vi "Header Table.vi"(5 "Cell Configuration":T1={"Cell Defaults"={"Background Color"=16777215, "Horizontal Align"=3, "Vertical Align"=1, "Minimum Height"=0.0, "Fixed Height"=0.0, "Padding"={"Left"=2.0, "Top"=2.0, "Right"=2.0, "Bottom"=3.0}}, "Borders"={"Left"={"Enabled"=FALSE, "Width"=1.0, "Color"=0}, "Top"={"Enabled"=FALSE, "Width"=1.0, "Color"=0}, "Right"={"Enabled"=FALSE, "Width"=1.0, "Color"=0}, "Bottom"={"Enabled"=FALSE, "Width"=1.0, "Color"=0}}, "Column Span"=0} {"Cell Defaults"."Vertical Align" items=["Bottom", "Middle", "Top"]; "Cell Defaults"."Horizontal Align" items=["Center", "Justified", "JustifiedAll", "Left", "Right"]}, 6 "Font":T6={"Font"="Arial", "Size"=10, "Colour"=0, "Bold"=FALSE, "Italic"=FALSE, "Underline"=FALSE, "Strikethrough"=FALSE, "Font Encoding"=enum."Cp1252, WinANSI"}, 7 "Table Configuration":T4={"Table Settings"={"Number of Columns"=2, "Width (%)"=100.0, "Relative Column Widths (%)"=[50.0, 50.0], "Horizontal Align"=0, "Header Rows"=0}, "Cell Defaults"={"Background Color"=16777215, "Horizontal Align"=3, "Vertical Align"=1, "Minimum Height"=0.0, "Fixed Height"=0.0, "Padding"={"Left"=2.0, "Top"=2.0, "Right"=2.0, "Bottom"=3.0}}, "Borders"={"Left"={"Enabled"=FALSE, "Width"=1.0, "Color"=16777215}, "Top"={"Enabled"=FALSE, "Width"=1.0, "Color"=16777215}, "Right"={"Enabled"=FALSE, "Width"=1.0, "Color"=16777215}, "Bottom"={"Enabled"=FALSE, "Width"=1.0, "Color"=16777215}, "Middle Horizontal"={"Enabled"=FALSE, "Width"=0.5, "Color"=16777215}, "Middle Vertical"={"Enabled"=FALSE, "Width"=0.5, "Color"=16777215}}} {"Cell Defaults"."Vertical Align" items=["Bottom", "Middle", "Top"]; "Cell Defaults"."Horizontal Align" items=["Center", "Justified", "JustifiedAll", "Left", "Right"]; "Table Settings"."Horizontal Align" items=["Center"=0, "Left"=3, "Right"=4]}, 8 "error in":errorcluster, 9 "Column Ratio left":sgl[](array[numeric]), 10 "Table":string[][](array[string]), 11 "Context In":refnum<class "Context.lvclass">=refnum) -> (0 "error out":errorcluster, 3 "Context Out":refnum<class "Context.lvclass">)   [LabVIEW 2020, in "PDF Interface.lvlib" / "PDF Interface Helper.lvlib"]
uses:
  PDF Interface Helper.lvlib
  <vilib>/Simplicity AI/SAI_PDF_API/Classes/Context/Controls/SAI_PDF_Font.ctl
  <vilib>/Simplicity AI/SAI_PDF_API/Classes/Context/Controls/SAI_PDF_Font Encoding.ctl
  <vilib>/Simplicity AI/SAI_PDF_API/Classes/Table Builder/Controls/SAI_PDF_Table Configuration.ctl
  <vilib>/Simplicity AI/SAI_PDF_API/Classes/Table Builder/Controls/SAI_PDF_Table Horizontal Align.ctl
  <vilib>/Simplicity AI/SAI_PDF_API/Classes/Table Builder/Controls/SAI_PDF_Default Cell Format.ctl
  <vilib>/Simplicity AI/SAI_PDF_API/Classes/Table Builder/Controls/SAI_PDF_BorderLine.ctl
  <vilib>/Simplicity AI/SAI_PDF_API/Classes/Table Builder/Controls/SAI_PDF_Cell Configuration.ctl
  <vilib>/Simplicity AI/SAI_PDF_API/Classes/Context/Context.lvclass
  <vilib>/Simplicity AI/SAI_PDF_API/Classes/Table Builder/Table Builder.lvclass
  Linearisierung V2/SpanEinstellungen/SpanEinstellungen.lvlib
panel:
  # "(Cp1252)"
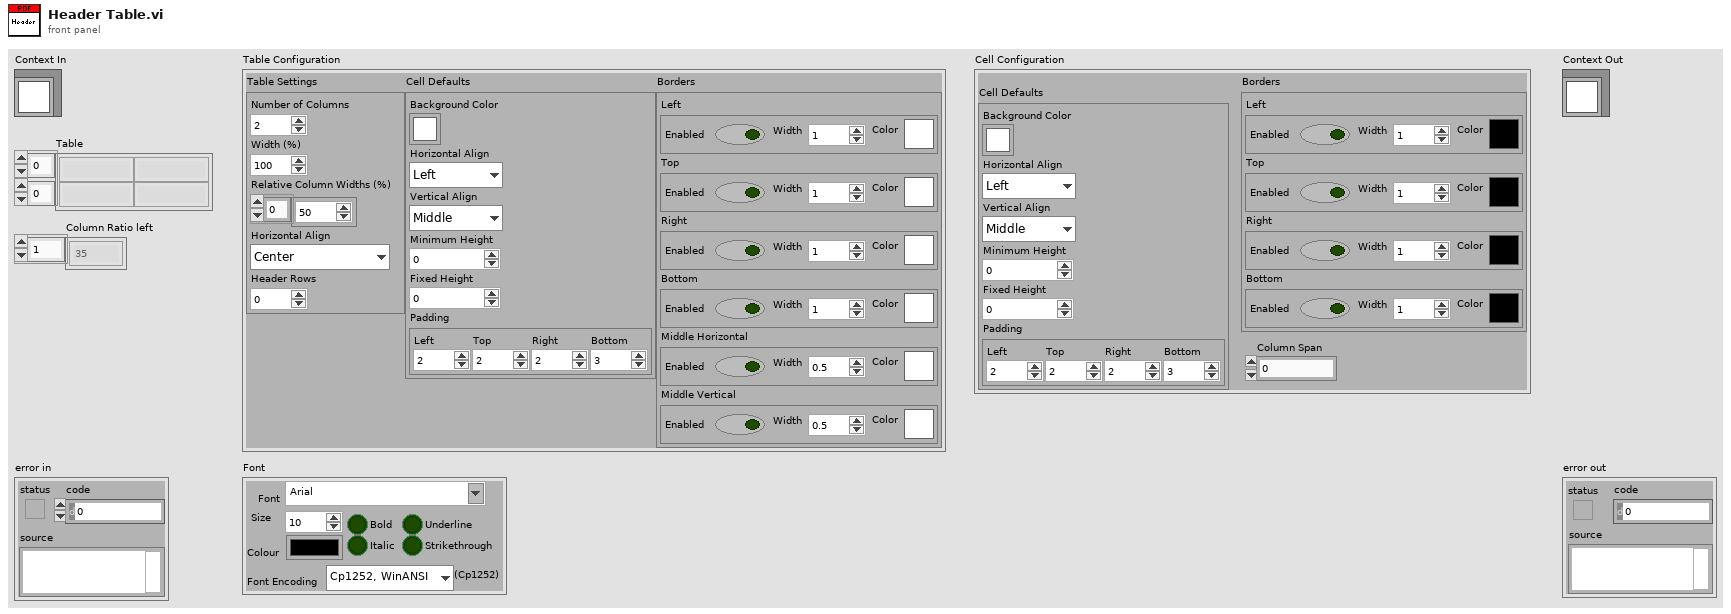
[diagram p1: front panel]
types:
  T1 = typedef "SAI_PDF_Toolkit.lvlib/Table Builder.lvclass/SAI_PDF_Cell Configuration.ctl" = cluster{"Cell Defaults":T2, "Borders":cluster{"Left":T3, "Top":T3, "Right":T3, "Bottom":T3}, "Column Span":i32}
  T2 = typedef "SAI_PDF_Toolkit.lvlib/Table Builder.lvclass/SAI_PDF_Default Cell Format.ctl" = cluster{"Background Color":u32, "Horizontal Align":i32, "Vertical Align":i32, "Minimum Height":sgl, "Fixed Height":sgl, "Padding":cluster{"Left":sgl, "Top":sgl, "Right":sgl, "Bottom":sgl}}
  T3 = typedef "SAI_PDF_Toolkit.lvlib/Table Builder.lvclass/SAI_PDF_BorderLine.ctl" = cluster{"Enabled":bool, "Width":sgl, "Color":u32}
  T4 = typedef "SAI_PDF_Toolkit.lvlib/Table Builder.lvclass/SAI_PDF_Table Configuration.ctl" = cluster{"Table Settings":cluster{"Number of Columns":i32, "Width (%)":sgl, "Relative Column Widths (%)":sgl[], "Horizontal Align":T5, "Header Rows":i32}, "Cell Defaults":T2, "Borders":cluster{"Left":T3, "Top":T3, "Right":T3, "Bottom":T3, "Middle Horizontal":T3, "Middle Vertical":T3}}
  T5 = typedef "SAI_PDF_Toolkit.lvlib/Table Builder.lvclass/SAI_PDF_Table Horizontal Align.ctl" = i32
  T6 = typedef "SAI_PDF_Toolkit.lvlib/Context.lvclass/SAI_PDF_Font.ctl" = cluster{"Font":string, "Size":i32, "Colour":u32, "Bold":bool, "Italic":bool, "Underline":bool, "Strikethrough":bool, "Font Encoding":T7}
  T7 = typedef "SAI_PDF_Toolkit.lvlib/Context.lvclass/SAI_PDF_Font Encoding.ctl" = enum16{"Cp1252, WinANSI", "IdentityH", "IdentityV", "Cp1250", "Cp1257", "MacRoman"}
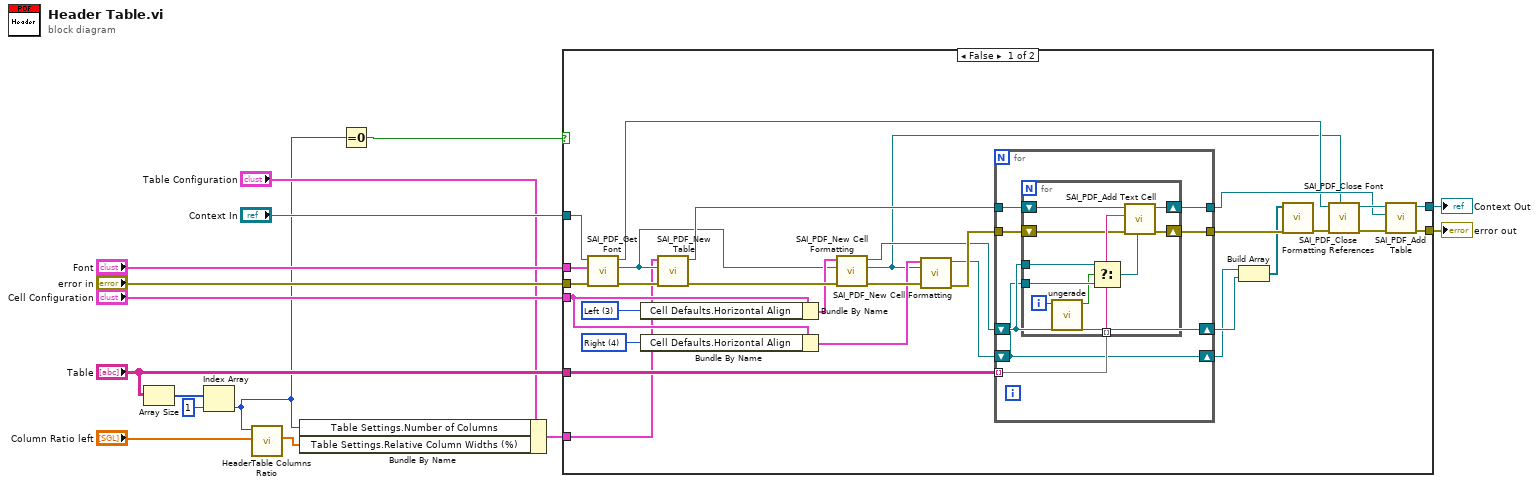
[diagram p0: block diagram]
diagram:
  n1 = Array Size(array="Table") -> (size(s)=w8:i32[])
  n2 = Index Array(array=w8, index=1 ("Index")) -> (element=w2:i32)
  n3 = call "HeaderTable Columns Ratio.vi"("Ratio left"="Column Ratio left", "Numerisch"=w2) -> ("Array ratio"=w4:sgl[])  [unwired: 8 in, 1 out]
  n4 = Bundle By Name(cluster="Table Configuration", "Table Settings.Number of Columns"=w2, "Table Settings.Relative Column Widths (%)"=w4) -> (w5:T4)
  n5 = Equal To 0?(x=w2) -> (x = 0?=w1:bool)
  n6 = case shown="False" w1 {
    tunnel: "Font" -> [w44 _]
    tunnel: "error in" -> [w43 w62]
    tunnel: "Context In" -> [w42 w63]
    tunnel: "Cell Configuration" -> [w36 _]
    tunnel: [w20 w63] -> w11
    tunnel: [w19 w62] -> w10
    tunnel: "Table" -> [w17 _]
    tunnel: w5 -> [w16 _]
    frame False {
      w40 = 4 items=["Center", "Justified", "JustifiedAll", "Left", "Right"] ("Horizontal Align")
      w39 = 3 items=["Center", "Justified", "JustifiedAll", "Left", "Right"] ("Horizontal Align")
      n7 = call <vilib>:"SAI_PDF_Get Font.vi"("error in"=w43, "Font"=w44, "Context In"=w42) -> ("error out"=w41:errorcluster, "Font"=w18:refnum<class "Font.lvclass">, "Context Out"=w21:refnum<class "Context.lvclass">)  [unwired: 6 out]
      n8 = Bundle By Name(cluster=w36, "Cell Defaults.Horizontal Align"=w39) -> (w37:T1)
      n9 = Bundle By Name(cluster=w36, "Cell Defaults.Horizontal Align"=w40) -> (w34:T1)
      n10 = call <vilib>:"SAI_PDF_New Table.vi"("error in"=w41, "Font In"=w18, "Table Configuration"=w16) -> ("error out"=w38:errorcluster, "Table Builder"=w33:refnum<class "Table Builder.lvclass">)  [unwired: 7 out]
      n11 = call <vilib>:"SAI_PDF_New Cell Formatting.vi"("error in"=w38, "Font In"=w18, "Cell Configuration"=w37) -> ("error out"=w35:errorcluster, "Cell Formatting"=w25:refnum<class "Formatting.lvclass">)  [unwired: 7 out]
      n12 = call <vilib>:"SAI_PDF_New Cell Formatting.vi"("error in"=w35, "Font In"=w18, "Cell Configuration"=w34) -> ("error out"=w32:errorcluster, "Cell Formatting"=w24:refnum<class "Formatting.lvclass">)  [unwired: 7 out]
      n13 = for {
        tunnel: w33 -> [w51]
        tunnel: w32 -> [w48]
        tunnel: [w47] -> w28
        tunnel: [w50] -> w22
        tunnel: w17 -> [w49] mode=indexing
        shift-right: [w46] -> w27
        shift-left: w25 -> [w46]
        shift-right: [w45] -> w26
        shift-left: w24 -> [w45]
        n14 = for {
          tunnel: w49 -> [w59] mode=indexing
          tunnel: w46 -> [w56]
          shift-right: [w60] -> w50
          shift-left: w51 -> [w61]
          shift-right: [w57] -> w47
          shift-left: w48 -> [w58]
          tunnel: w45 -> [w55]
          i -> [w53]
          n15 = call "ungerade.vi"("Zahl"=w53) -> ("ungerade ?"=w52:bool)  [unwired: 10 in]
          n16 = Select(t=w56, s=w52, f=w55) -> (s? t:f=w54:refnum<class "Formatting.lvclass">)
          n17 = call <vilib>:"SAI_PDF_Add Text Cell.vi"("Formatting In"=w54, "error in"=w58, "Text"=w59, "Table Builder In"=w61) -> ("error out"=w57:errorcluster, "Table Builder Out"=w60:refnum<class "Table Builder.lvclass">)  [unwired: 6 in]
        }
      }
      n18 = Build Array(w26, w27) -> (w23:refnum<class "Formatting.lvclass">[])
      n19 = call <vilib>:"SAI_PDF_Close Formatting References.vi"("error in"=w28, "Formatting Refs"=w23) -> ("error out"=w29:errorcluster)  [unwired: 9 out]
      n20 = call <vilib>:"SAI_PDF_Close Font.vi"("Font"=w18, "error in"=w29, "Context In"=w21) -> ("error out"=w30:errorcluster, "Context Out"=w31:refnum<class "Context.lvclass">)  [unwired: 7 out]
      n21 = call <vilib>:"SAI_PDF_Add Table.vi"("error in"=w30, "Table Builder In"=w22, "Context In"=w31) -> ("error out"=w19:errorcluster, "Context Out"=w20:refnum<class "Context.lvclass">)  [unwired: 7 out]
    }
    frame True {
    }
  }
  "error out" <- w10
  "Context Out" <- w11
